vi "ViHandler.UnRegisterVi.vi"(8 "error in (no error)":errorcluster, 10 "ViInfo":T1, 11 "ViHandler in":refnum<class "ViHandler.lvclass">) -> (0 "error out":errorcluster, 2 "UnregisterSuccessful?":bool, 3 "ViHandler out":refnum<class "ViHandler.lvclass">)   [LabVIEW 2016, in "ViHandler.lvclass"]
uses:
  ViHandler.lvclass
  ViHandler.ViInfo.ctl
  ViHandler.lvclass/ViHandler.ctl
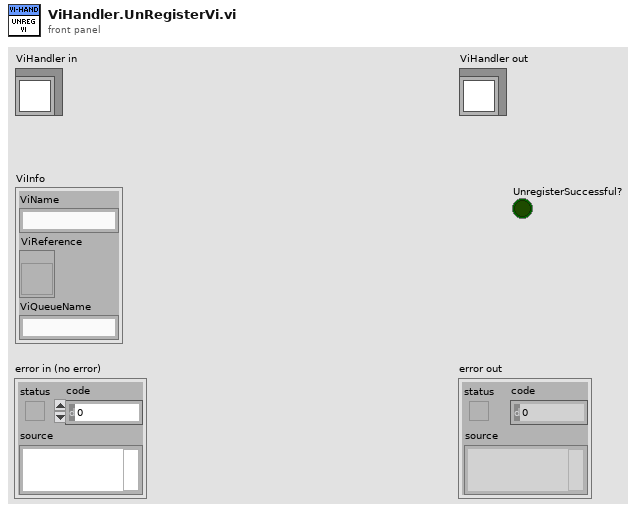
[diagram p1: front panel]
types:
  T1 = typedef "ViHandler.lvclass/ViHandler.ViInfo.ctl" = cluster{"ViName":string, "ViReference":refnum<vi>, "ViQueueName":string}
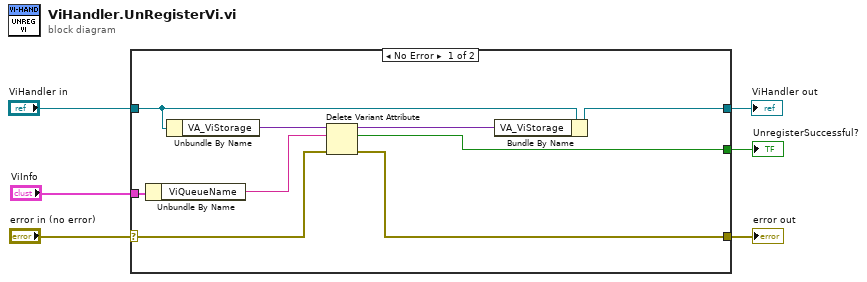
[diagram p0: block diagram]
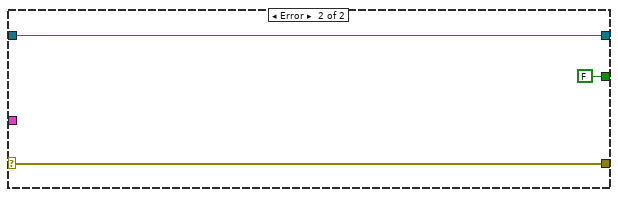
[diagram p2: hidden frame]
diagram:
  n1 = case shown="No Error" "error in (no error)" {
    selector: "error in (no error)" -> [w11 w18]
    tunnel: [w10 w18] -> w5
    tunnel: [w9 w17] -> w3
    tunnel: "ViHandler in" -> [w14 w17]
    tunnel: "ViInfo" -> [w15 _]
    tunnel: [w7 FALSE ("found")] -> w1
    frame No Error {
      n2 = Unbundle By Name(w15) -> ("ViQueueName"=w12:string)
      n3 = Unbundle By Name(w14) -> ("VA_ViStorage"=w13:variant)
      n4 = Delete Variant Attribute(4:w11, 6:w12, 7:w13) -> (0:w10:errorcluster, 2:w7:bool, 3:w8:variant)
      n5 = Bundle By Name(cluster=w14, "VA_ViStorage"=w8) -> (w9:refnum<class "ViHandler.lvclass">)
    }
    frame Error {
    }
  }
  "error out" <- w5
  "ViHandler out" <- w3
  "UnregisterSuccessful?" <- w1
